vi "Disable Embedded Data Logger Custom Device.vi"(8 "error in":errorcluster, 11 "embedded data logger in":T1 format="%.0x") -> (0 "error out":errorcluster, 3 "embedded data logger out":T1 format="%.0x")   [LabVIEW 2027, in "Embedded Data Logger Scripting.lvlib"]
uses:
  Embedded Data Logger Scripting.lvlib
  <vilib>/NI VeriStand/Custom Device API/Custom Device API.lvlib
  Shared/Constants.vi
  Shared/Embedded Data Logger Shared.lvlib
  C:/NetCore/niveristand-embedded-data-logger-custom-device/Source/Scripting/Custom Device/Disable Embedded Data Logger Custom Device.vi/NationalInstruments.VeriStand.SystemDefinitionAPI
  NationalInstruments.VeriStand.SystemDefinitionAPI
  <vilib>/NI VeriStand/Custom Device API/Custom Device Item Ref.ctl
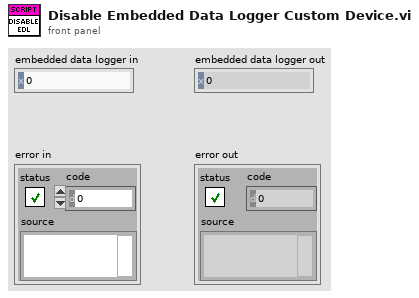
[diagram p1: front panel]
types:
  T1 = typedef "Custom Device API.lvlib/Custom Device Item Ref.ctl" = u64
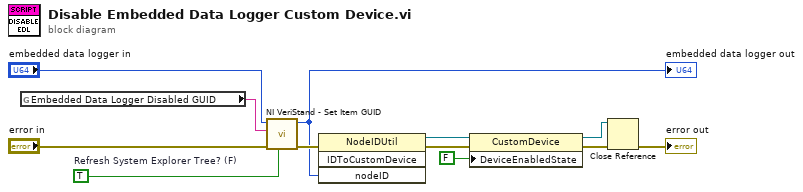
[diagram p0: block diagram]
diagram:
  w12 = TRUE  # Refresh System Explorer Tree? (F)
  n1 = global read "Constants.vi" "Embedded Data Logger Disabled GUID"() -> (w11:string)
  n2 = call <vilib>:"NI VeriStand - Set Item GUID.vi"("Refresh System Explorer Tree? (F)"=w12, "error in (no error)"="error in", "GUID"=w11, "Item Ref in"="embedded data logger in") -> ("error out"=w8:errorcluster, "Item Ref out"=w1:T1)  [unwired: 6 in]
  "embedded data logger out" <- w1
  n3 = invoke class="NodeIDUtil" method="IDToCustomDevice"(error in=w8, "nodeID"=w1) -> (error out=w5:errorcluster, "IDToCustomDevice"=w7:refnum<k39>)  [unwired: 2 in, 2 out]
  n4 = property class="CustomDevice"(reference=w7, error in=w5, "DeviceEnabledState"=FALSE) -> (reference out=w2:refnum<k39>, error out=w4:errorcluster)
  n5 = Close Reference(reference=w2, error in (no error)=w4) -> (error out=→"error out":errorcluster)
